vi "GetDataSetRegistration.vi"(8 "error in (no error)":errorcluster, 10 "data group name":string, 11 "virtual channel config":T1) -> (0 "error out":errorcluster, 1 "atleast one data set to register":bool, 2 "register data set":T3)   [LabVIEW 2017, in "McsaVirtualChannel.lvlib"]
uses:
  <vilib>/addons/InsightCM/Devices/Shared/Mcsa/McsaVirtualChannel/McsaVirtualChannel.lvlib
  <vilib>/addons/InsightCM/Devices/Shared/Mcsa/McsaDataEventCreator/controls/RegisterDataSets.ctl
  <vilib>/addons/InsightCM/Devices/Shared/Mcsa/McsaDataEventCreator/controls/Registry_DataSet.ctl
  <vilib>/addons/InsightCM/Devices/Shared/Mcsa/McsaDataEventCreator/controls/DataSetType.ctl
  <vilib>/addons/InsightCM/Devices/Shared/Mcsa/McsaVirtualChannel/controls/VirtualChannelGroup.ctl
  <vilib>/addons/InsightCM/Devices/Shared/Mcsa/McsaVirtualChannel/controls/VirtualChannel.ctl
  <vilib>/addons/InsightCM/Devices/Shared/Mcsa/McsaDataEventCreator/McsaDataEventCreator.lvlib
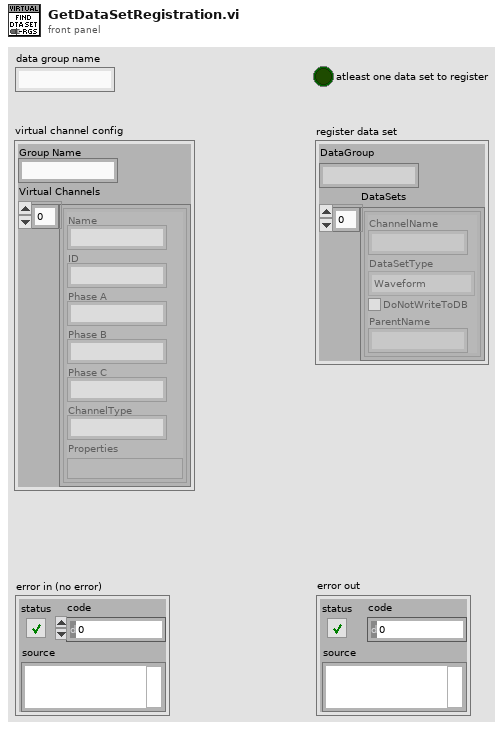
[diagram p1: front panel]
types:
  T1 = typedef "McsaVirtualChannel.lvlib/VirtualChannelGroup.ctl" = cluster{"Group Name":string, "Virtual Channels":T2[]}
  T2 = typedef "McsaVirtualChannel.lvlib/VirtualChannel.ctl" = cluster{"Name":string, "ID":string, "Phase A":string, "Phase B":string, "Phase C":string, "ChannelType":string, "Properties":variant}
  T3 = typedef "McsaDataEventCreator.lvlib/RegisterDataSets.ctl" = cluster{"DataGroup":string, "DataSets":T4[]}
  T4 = typedef "McsaDataEventCreator.lvlib/Registry_DataSet.ctl" = cluster{"ChannelName":string, "DataSetType":T5, "DoNotWriteToDB":bool, "ParentName":string}
  T5 = typedef "McsaDataEventCreator.lvlib/DataSetType.ctl" = enum16{"Waveform", "MCSAFFT", "TorqueWFM"}
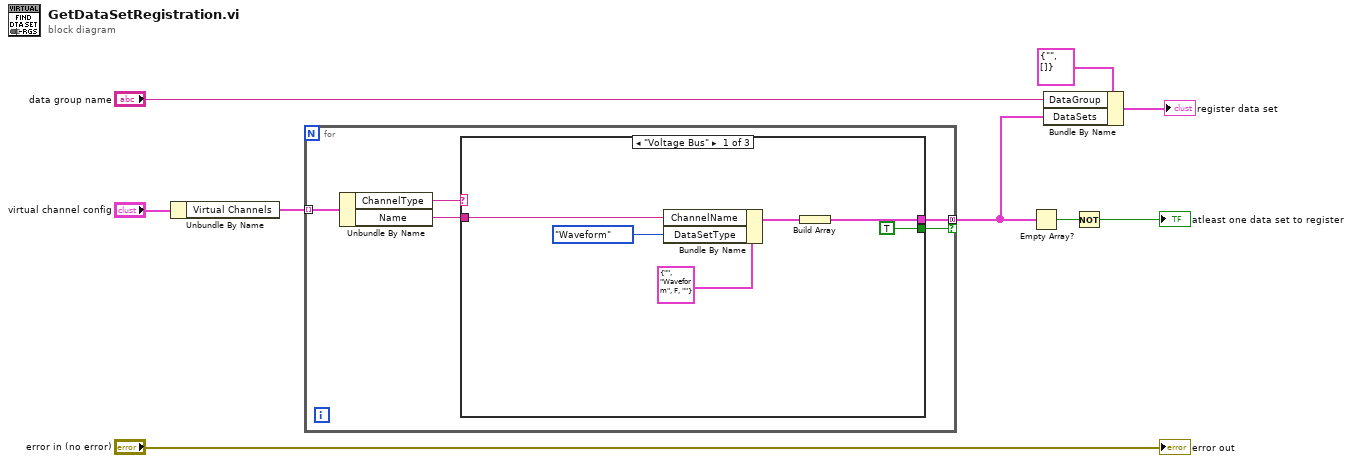
[diagram p0: block diagram]
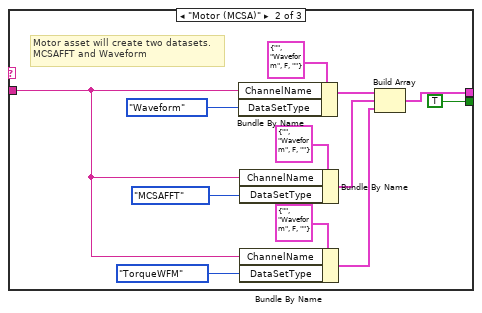
[diagram p2: hidden frame]
diagram:
  n1 = Unbundle By Name("virtual channel config") -> ("Virtual Channels"=w1:T2[])
  n2 = for {
    tunnel: [w10] -> w8 mode=concatenating if=w14
    tunnel: w1 -> [w13] mode=indexing
    n3 = Unbundle By Name(w13) -> ("ChannelType"=w12:string, "Name"=w11:string)
    n4 = case shown="\"Voltage Bus\"" w12 {
      tunnel: w11 -> [w20 w23 _]
      tunnel: [TRUE TRUE _] -> w14
      tunnel: [w17 w30 _] -> w10
      frame "Voltage Bus" {
        n5 = Bundle By Name(cluster=T4 {"ChannelName"="", "DataSetType"=enum."Waveform", "DoNotWriteToDB"=FALSE, "ParentName"=""} ("DataSet"), "ChannelName"=w20, "DataSetType"=DataSetType."Waveform") -> (w18:T4)
        n6 = Build Array(w18) -> (w17:T4[])
      }
      frame "Motor (MCSA)" {
        # "Motor asset will create two datasets.\nMCSAFFT and Waveform"
        n7 = Bundle By Name(cluster=T4 {"ChannelName"="", "DataSetType"=enum."Waveform", "DoNotWriteToDB"=FALSE, "ParentName"=""} ("DataSet"), "ChannelName"=w23, "DataSetType"=DataSetType."Waveform") -> (w31:T4)
        n8 = Bundle By Name(cluster=T4 {"ChannelName"="", "DataSetType"=enum."Waveform", "DoNotWriteToDB"=FALSE, "ParentName"=""} ("DataSet"), "ChannelName"=w23, "DataSetType"=DataSetType."MCSAFFT") -> (w29:T4)
        n9 = Bundle By Name(cluster=T4 {"ChannelName"="", "DataSetType"=enum."Waveform", "DoNotWriteToDB"=FALSE, "ParentName"=""} ("DataSet"), "ChannelName"=w23, "DataSetType"=DataSetType."TorqueWFM") -> (w21:T4)
        n10 = Build Array(w31, w29, w21) -> (w30:T4[])
      }
      frame Default {
      }
    }
  }
  n11 = Empty Array?(array=w8) -> (empty?=w7:bool)
  n12 = Bundle By Name(cluster=T3 {"DataGroup"="", "DataSets"=[]} ("RegisterDataSet"), "DataGroup"="data group name", "DataSets"=w8) -> (→"register data set":T3)
  n13 = Not(x=w7) -> (.not. x?=→"atleast one data set to register":bool)
  "error out" <- "error in (no error)"
